vi "Main IU.vi"() -> ()   [LabVIEW 2018]
uses:
  <vilib>/Analysis/baseanly.llb/Mean (DBL).vi
  <vilib>/Utility/file.llb/Read Delimited Spreadsheet (DBL).vi
  <vilib>/Analysis/NI_AALBase.lvlib
panel:
  in  "Escriba el tiempo para ejecutar\ntrayectoria suave":dbl
  in  "Setpoint 2":dbl
  in  "Setpoint 1":dbl
  in  "Homing":bool
  out "EsfuerzoSat 2":dbl(graph)
  out "SetpointVsSalida 2":cluster{"Double":dbl, "Output":dbl}(graph)
  out "EsfuerzoSat":dbl(graph)
  out "SetpointVsSalida":cluster{"Double":dbl, "Output":dbl}(graph)
  out "Saving Data":bool
  in  "Record Button":bool
  in  "Filename":path=path "test.lvm"
  out "Motor1":waveform(dbl)[](graph)
  in  "Paro Emergencia:\nUI y RT":bool
  in  "Stop UI":bool
  # "s"
  # "Esta automáticamente se ejecutará"
  # "rad/s^2"
  # "rad/s^2"
  # "rad"
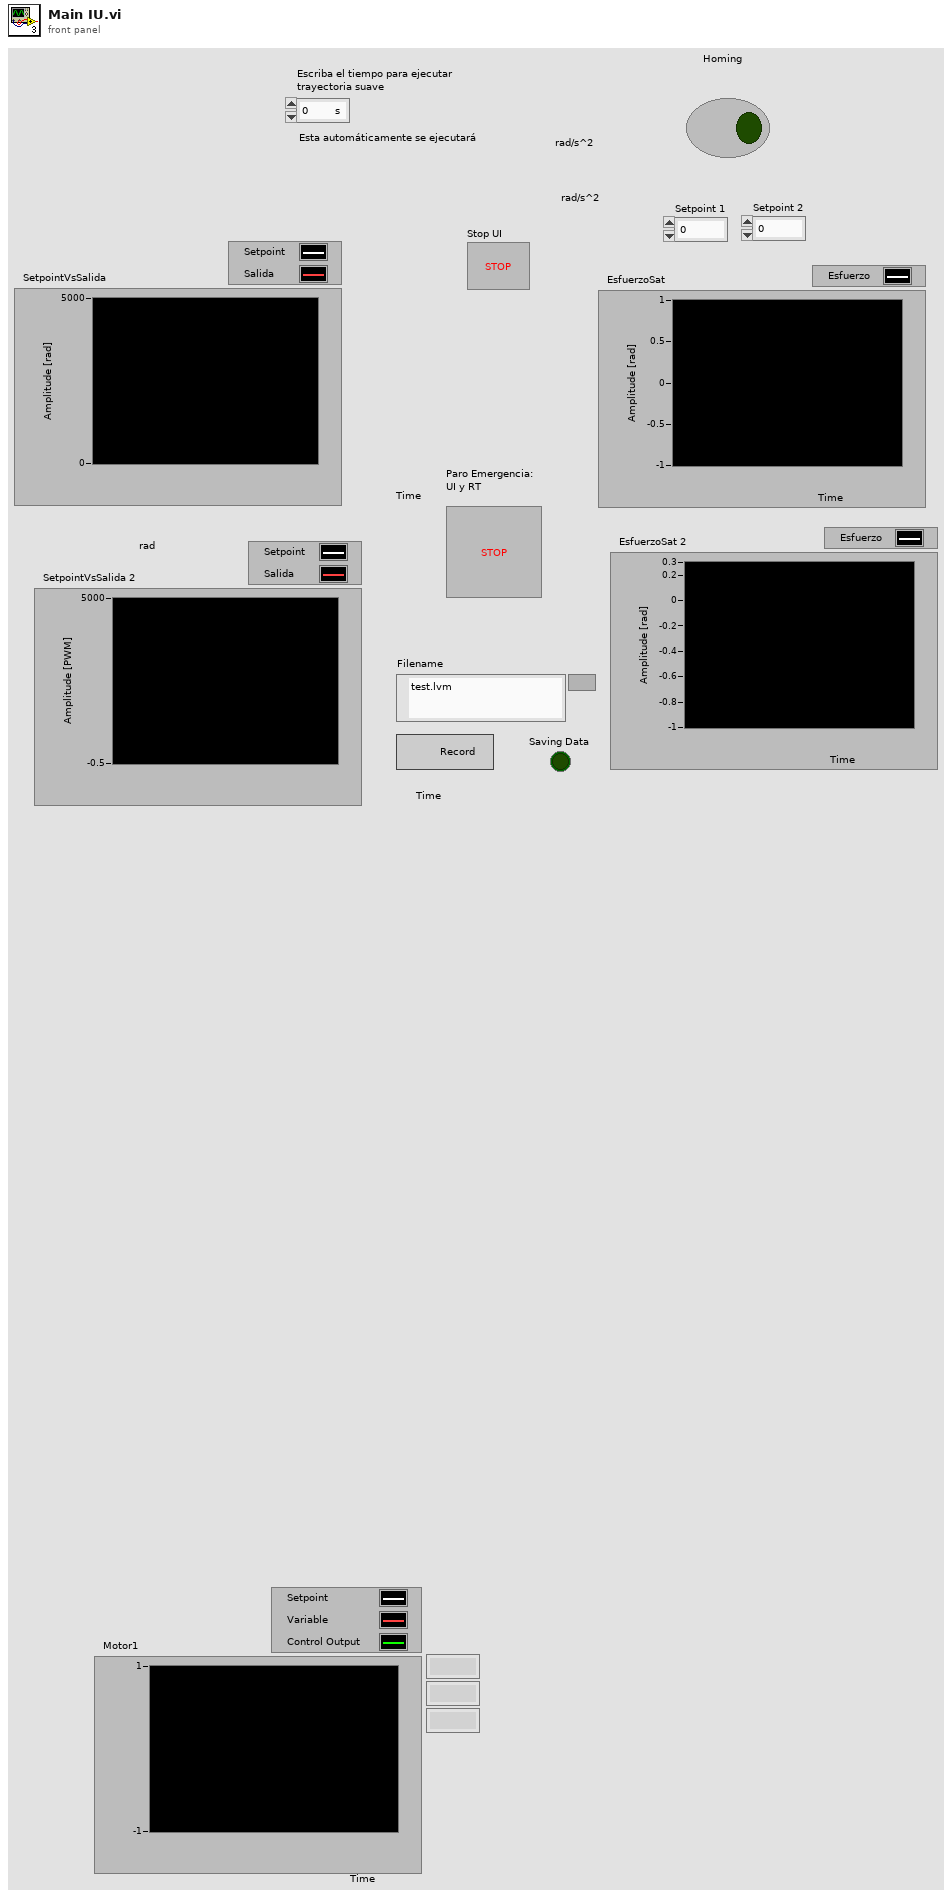
[diagram p1: front panel]
types:
  T1 = cluster{"Double":dbl, "dbl Scaled Value":dbl, "Output":dbl, "seconds since 1Jan1904":timestamp, dbl, dbl, dbl}
  T2 = cluster{"writer name":string, "Variant":variant, "Variant":variant}
  T3 = cluster{"Double":dbl, "dbl Scaled Value":dbl, "Output":dbl, "seconds since 1Jan1904":timestamp, dbl, dbl, dbl}[]
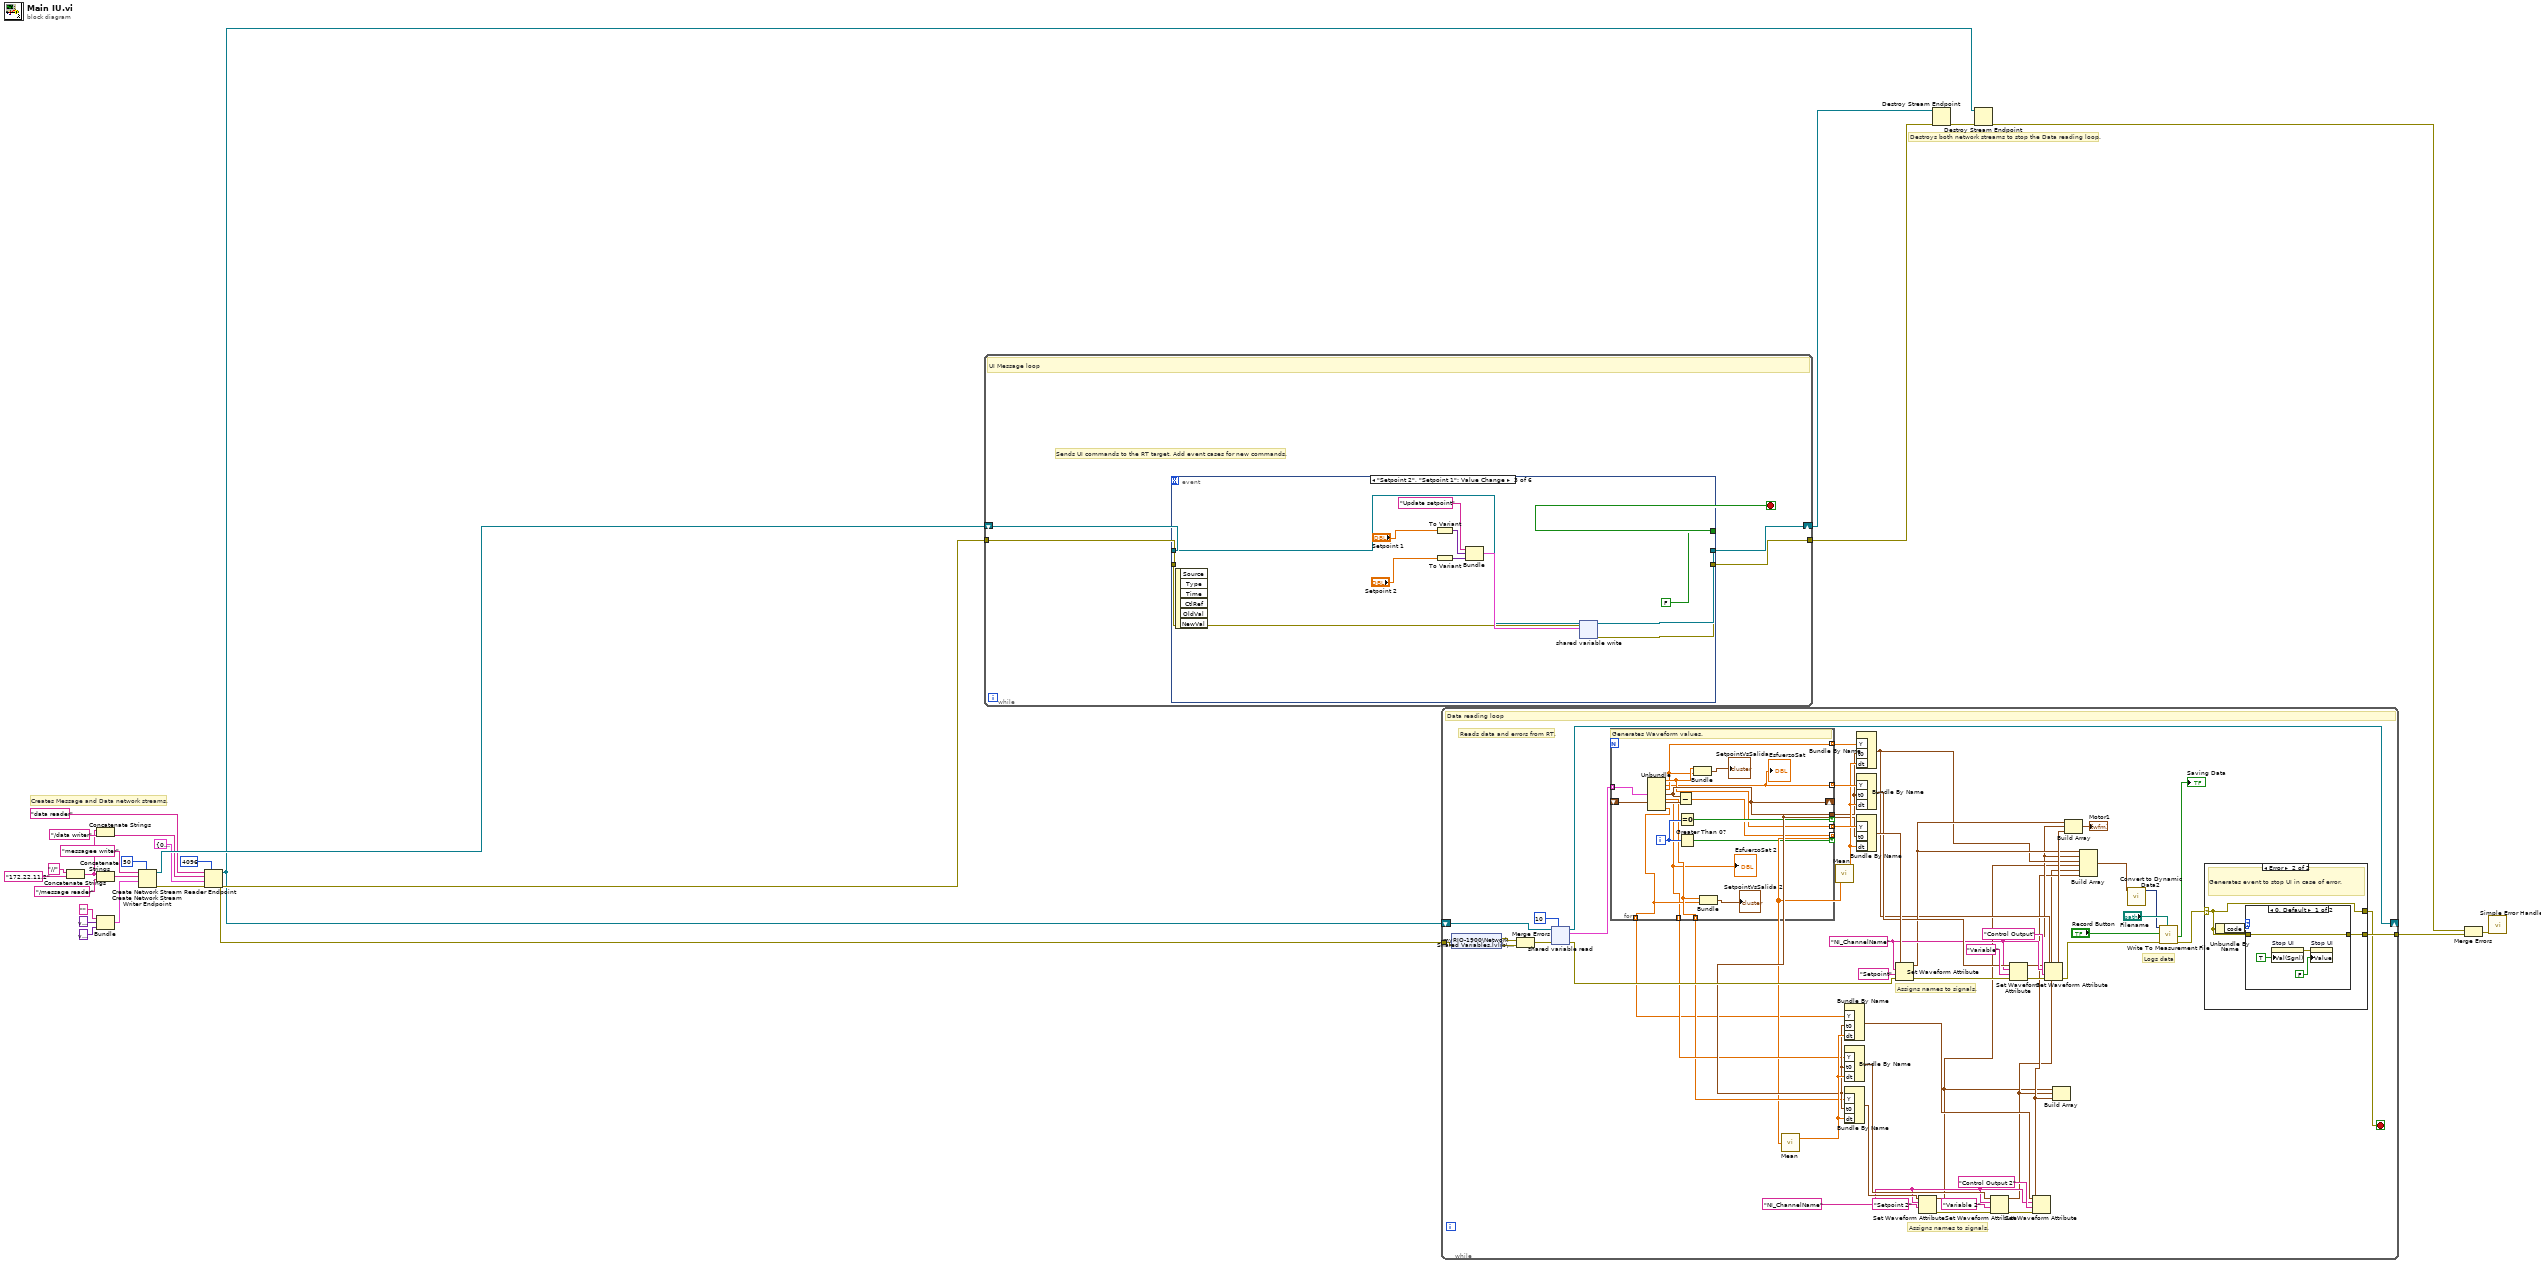
[diagram p0: block diagram]
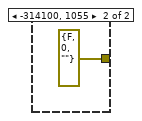
[diagram p3: hidden frame]
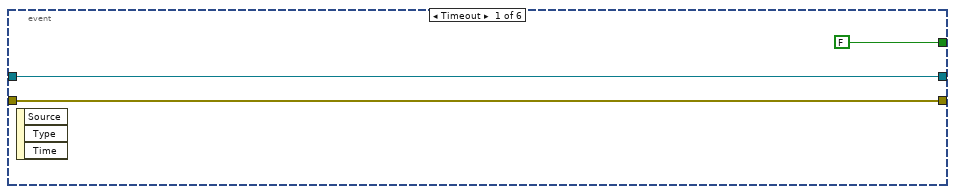
[diagram p4: hidden frame]
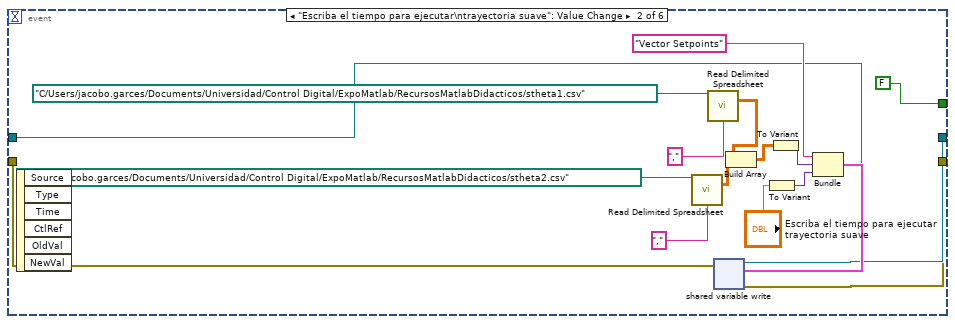
[diagram p5: hidden frame]
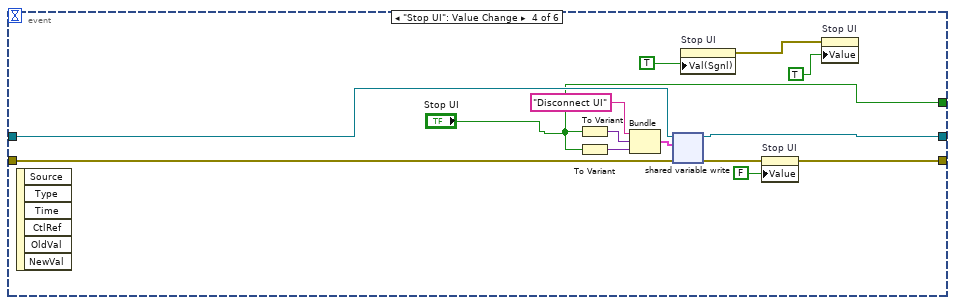
[diagram p6: hidden frame]
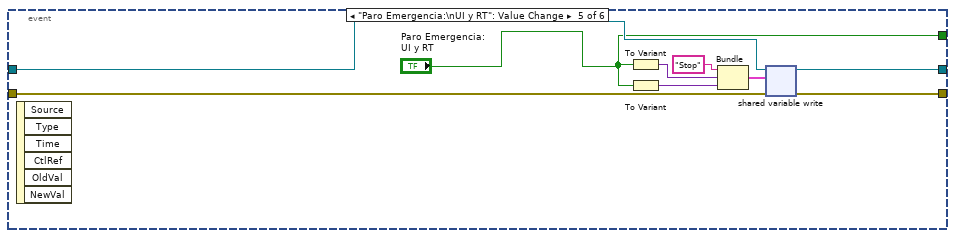
[diagram p7: hidden frame]
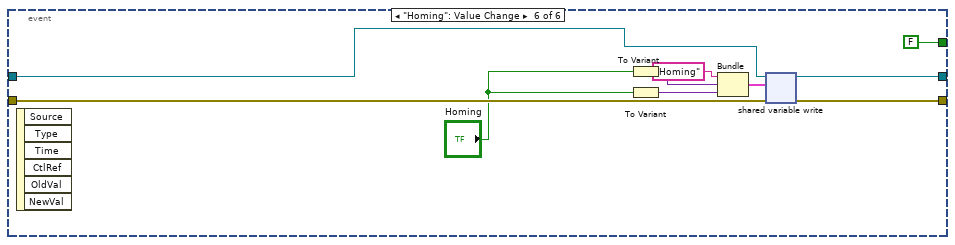
[diagram p8: hidden frame]
diagram:
  # "Destroys both network streams to stop the Data reading loop."
  # "Creates Message and Data network streams."
  n1 = Concatenate Strings("//", "172.22.11.2" ("myRIO IP")) -> (w2:string)
  n2 = Bundle("", variant, variant) -> (w26:cluster{string, variant, variant})  [unwired: 1 in]
  n3 = Concatenate Strings(w2, "/data writer") -> (w17:string)
  n4 = Concatenate Strings(w2, "/message reader") -> (w3:string)
  n5 = Create Network Stream Writer Endpoint(7:50 ("writer buffer size"), 9:w26, 10:w3, 11:"messagee writer" ("writer name")) -> (0:w14:errorcluster, 3:w20:refnum<k21>)  [unwired: 3 in]
  n6 = Create Network Stream Reader Endpoint(7:4096 ("reader buffer size"), 8:w14, 9:T1 {"Double"=0.0, "dbl Scaled Value"=0.0, "Output"=0.0, "seconds since 1Jan1904"=timestamp(0 s since 1904-01-01), 0.0, 0.0, 0.0} ("Data"), 10:w17, 11:"data reader" ("reader name")) -> (0:w13:errorcluster, 3:w6:refnum<k21>)  [unwired: 2 in]
  n7 = while {
    tunnel: w13 -> [w27]
    shift-right: [w31] -> w8
    shift-left: w20 -> [w28]
    tunnel: [w30] -> w9
    stop <- w29 stop-if-true
    # "Sends UI commands to the RT target. Add event cases for new commands."
    # "UI Message loop"
    n8 = event shown="[2] \"Setpoint 2\", \"Setpoint 1\": Value Change" {
      selector: _ -> [_ _ _ _ _ _]
      dyn-events: _ -> [_ _ _ _ _ _]
      timeout: _ -> [_ _ _ _ _ _]
      tunnel: [w33 w46 w57 w73 w81 w91] -> w31
      tunnel: [w32 w45 w56 w70 w82 w92] -> w30
      tunnel: [FALSE ("Stop UI and RT") FALSE ("Stop UI and RT") FALSE ("Stop UI and RT") "Stop UI" "Paro Emergencia:\nUI y RT" FALSE] -> w29
      tunnel: w28 -> [w33 w44 w55 w67 w79 w89]
      tunnel: w27 -> [w32 w43 w54 w68 w78 w88]
      event Timeout {
        n9 = event-data() -> ()  [unwired: 1 in, 3 out]
      }
      event "Escriba el tiempo para ejecutar\ntrayectoria suave": Value Change {
        n10 = event-data() -> ()  [unwired: 1 in, 6 out]
        n11 = call-poly <vilib>:"Read Delimited Spreadsheet.vi"("file path (dialog if empty)"=path "C:/Users/jacobo.garces/Documents/Universidad/Control Digital/ExpoMatlab/RecursosMatlabDidacticos/stheta2.csv", "delimiter (\\t)"="," ("delimiter (\\t)")) -> ("all rows"=w38:dbl[][])  [unwired: 8 in, 5 out]
        n12 = call-poly <vilib>:"Read Delimited Spreadsheet.vi"("file path (dialog if empty)"=path "C:/Users/jacobo.garces/Documents/Universidad/Control Digital/ExpoMatlab/RecursosMatlabDidacticos/stheta1.csv", "delimiter (\\t)"="," ("delimiter (\\t)")) -> ("all rows"=w37:dbl[][])  [unwired: 8 in, 5 out]
        n13 = Build Array(w37, w38) -> (w36:dbl[][][])
        n14 = To Variant(anything="Escriba el tiempo para ejecutar\ntrayectoria suave") -> (Variant=w49:variant)
        n15 = To Variant(anything=w36) -> (Variant=w47:variant)
        n16 = Bundle("writer name"="Vector Setpoints", "Variant"=w47, "Variant"=w49) -> (w48:T2)  [unwired: 1 in]
        n17 = shared-variable-write(w44, w43, w48) -> (w46:refnum<k21>, w45:errorcluster)  [unwired: 1 in, 1 out]
      }
      event "Setpoint 2", "Setpoint 1": Value Change {
        n18 = event-data() -> ()  [unwired: 1 in, 6 out]
        n19 = To Variant(anything="Setpoint 1") -> (Variant=w58:variant)
        n20 = To Variant(anything="Setpoint 2") -> (Variant=w60:variant)
        n21 = Bundle("writer name"="Update setpoint", "Variant"=w58, "Variant"=w60) -> (w59:T2)  [unwired: 1 in]
        n22 = shared-variable-write(w55, w54, w59) -> (w57:refnum<k21>, w56:errorcluster)  [unwired: 1 in, 1 out]
      }
      event "Stop UI": Value Change {
        n23 = event-data() -> ()  [unwired: 1 in, 6 out]
        n24 = To Variant(anything="Stop UI") -> (Variant=w76:variant)
        n25 = To Variant(anything="Stop UI") -> (Variant=w69:variant)
        n26 = Bundle("writer name"="Disconnect UI", "Variant"=w76, "Variant"=w69) -> (w75:T2)  [unwired: 1 in]
        n27 = shared-variable-write(w67, w68, w75) -> (w73:refnum<k21>, w71:errorcluster)  [unwired: 1 in, 1 out]
        n28 = property on="Stop UI" class="Bool (strict)"("Val(Sgnl)"=TRUE ("Stop UI and RT")) -> (error out=w66:errorcluster)  [unwired: 2 in, 1 out]
        n29 = property on="Stop UI" class="Bool (strict)"(error in=w71, "Value"=FALSE ("Stop UI and RT")) -> (error out=w70:errorcluster)  [unwired: 1 in, 1 out]
        n30 = property on="Stop UI" class="Bool (strict)"(error in=w66, "Value"=TRUE ("Stop UI")) -> ()  [unwired: 1 in, 2 out]
      }
      event "Paro Emergencia:\nUI y RT": Value Change {
        n31 = event-data() -> ()  [unwired: 1 in, 6 out]
        n32 = To Variant(anything="Paro Emergencia:\nUI y RT") -> (Variant=w85:variant)
        n33 = To Variant(anything="Paro Emergencia:\nUI y RT") -> (Variant=w80:variant)
        n34 = Bundle("writer name"="Stop", "Variant"=w85, "Variant"=w80) -> (w84:T2)  [unwired: 1 in]
        n35 = shared-variable-write(w79, w78, w84) -> (w81:refnum<k21>, w82:errorcluster)  [unwired: 1 in, 1 out]
      }
      event "Homing": Value Change {
        n36 = event-data() -> ()  [unwired: 1 in, 6 out]
        n37 = To Variant(anything="Homing") -> (Variant=w95:variant)
        n38 = To Variant(anything="Homing") -> (Variant=w90:variant)
        n39 = Bundle("writer name"="Homing", "Variant"=w95, "Variant"=w90) -> (w94:T2)  [unwired: 1 in]
        n40 = shared-variable-write(w89, w88, w94) -> (w91:refnum<k21>, w92:errorcluster)  [unwired: 1 in, 1 out]
      }
    }
  }
  n41 = while {
    tunnel: w13 -> [w123]
    shift-right: [w133] -> _
    shift-left: w6 -> [w148]
    tunnel: [w122] -> w10
    stop <- w121 stop-if-true
    w110 = "NI_ChannelName" ("name")
    w127 = "NI_ChannelName" ("name")
    # "Assigns names to signals."
    # "Logs data"
    # "Assigns names to signals."
    # "Reads data and errors from RT."
    # "Data reading loop"
    n42 = shared-variable "myRIO-1900\\Network Shared Variables.lvlib\\error IO"(error in=w123) -> (w126:errorcluster, error out=w125:errorcluster)
    n43 = Merge Errors(w126, w125) -> (w124:errorcluster)
    n44 = shared-variable-read(w148, w124, 10 ("# elements")) -> (w133:refnum<k21>, w138:errorcluster, w146:T3)  [unwired: 1 in, 1 out]
    n45 = for {
      tunnel: w146 -> [w172] mode=indexing
      tunnel: [w165] -> w145 mode=indexing
      tunnel: [w162] -> w144 mode=indexing
      tunnel: [w164] -> w120 mode=indexing
      tunnel: [w170] -> w109 if=w171
      shift-right: [w170] -> _
      shift-left: _ -> [w169]
      tunnel: [w168] -> w106 mode=indexing if=w166
      tunnel: [w159] -> w105 mode=indexing
      tunnel: [w158] -> w108 mode=indexing
      tunnel: [w160] -> w107 mode=indexing
      i -> [w167]
      # "Generates Waveform values."
      n46 = Unbundle(w172) -> ("Double"=w165:dbl, "dbl Scaled Value"=w162:dbl, "Output"=w164:dbl, "seconds since 1Jan1904"=w170:timestamp, w160:dbl, w158:dbl, w159:dbl)
      "EsfuerzoSat" <- w162
      "EsfuerzoSat 2" <- w158
      n47 = Subtract(x=w170, y=w169) -> (x-y=w168:dbl)
      n48 = Equal To 0?(x=w167) -> (x = 0?=w171:bool)
      n49 = Greater Than 0?(x=w167) -> (x > 0?=w166:bool)
      n50 = Bundle("Double"=w165, "Output"=w164) -> (→"SetpointVsSalida":cluster{"Double":dbl, "Output":dbl})  [unwired: 1 in]
      n51 = Bundle(w160, w159) -> (→"SetpointVsSalida 2":cluster{dbl, dbl})  [unwired: 1 in]
    }
    n52 = call-poly <vilib>:"Mean.vi"("X"=w106) -> ("mean"=w119:dbl)  [unwired: 1 out]
    n53 = call-poly <vilib>:"Mean.vi"("X"=w106) -> ("mean"=w143:dbl)  [unwired: 1 out]
    n54 = Bundle By Name("Y"=w105, "t0"=w109, "dt"=w119) -> (w111:waveform(dbl))  [unwired: 1 in]
    n55 = Bundle By Name("Y"=w108, "t0"=w109, "dt"=w119) -> (w112:waveform(dbl))  [unwired: 1 in]
    n56 = Bundle By Name("Y"=w107, "t0"=w109, "dt"=w119) -> (w118:waveform(dbl))  [unwired: 1 in]
    n57 = Bundle By Name("Y"=w120, "t0"=w109, "dt"=w143) -> (w101:waveform(dbl))  [unwired: 1 in]
    n58 = Bundle By Name("Y"=w144, "t0"=w109, "dt"=w143) -> (w135:waveform(dbl))  [unwired: 1 in]
    n59 = Bundle By Name("Y"=w145, "t0"=w109, "dt"=w143) -> (w142:waveform(dbl))  [unwired: 1 in]
    n60 = Set Waveform Attribute(4:w138, 5:"Setpoint" ("name"), 6:w127, 7:w142) -> (0:w137:errorcluster, 3:w102:waveform(dbl))  [unwired: 1 out]
    n61 = Set Waveform Attribute(5:"Setpoint 2" ("name"), 6:w110, 7:w118) -> (0:w114:errorcluster, 3:w97:waveform(dbl))  [unwired: 1 in, 1 out]
    n62 = Set Waveform Attribute(4:w114, 5:"Variable 2" ("name"), 6:w110, 7:w112) -> (0:w113:errorcluster, 3:w98:waveform(dbl))  [unwired: 1 out]
    n63 = Set Waveform Attribute(4:w137, 5:"Variable" ("name"), 6:w127, 7:w135) -> (0:w136:errorcluster, 3:w100:waveform(dbl))  [unwired: 1 out]
    n64 = Set Waveform Attribute(4:w113, 5:"Control Output 2" ("name"), 6:w110, 7:w111) -> (3:w99:waveform(dbl))  [unwired: 2 out]
    n65 = Set Waveform Attribute(4:w136, 5:"Control Output" ("name"), 6:w127, 7:w101) -> (0:w132:errorcluster, 3:w134:waveform(dbl))  [unwired: 1 out]
    n66 = Build Array(w97, w98, w99) -> ()  [unwired: 1 out]
    n67 = Build Array(w102, w100, w134) -> (→"Motor1":waveform(dbl)[])
    n68 = Build Array(w102, w100, w101, w97, w98, w99) -> (w96:waveform(dbl)[])
    n69 = call "Convert to Dynamic Data2"("Array of Waveforms"=w96) -> ("Dynamic Data Type"=w103:dynamicdata)  [unwired: 3 in]
    n70 = call "Write To Measurement File"("Signals"=w103, "Enable"="Record Button", "error in (no error)"=w132, "Filename"="Filename") -> ("Saving Data"=→"Saving Data":bool, "error out"=w128:errorcluster)  [unwired: 13 in, 1 out]
    n71 = case shown="Error" w128 {
      selector: w128 -> [w149 w150]
      tunnel: [w149 w151] -> w122
      tunnel: [w149 w150] -> w121
      frame No Error {
        # "No action required."
      }
      frame Error {
        # "Generates event to stop UI in case of error."
        n72 = Unbundle By Name(w150) -> ("code"=w152:i32)
        n73 = case shown="0, Default" w152 {
          tunnel: [w155 errorcluster {"status"=FALSE, "code"=0, "source"=""} ("error IO")] -> w151
          tunnel: w150 -> [w155 _]
          frame 0, Default {
            n74 = property on="Stop UI" class="Bool (strict)"("Val(Sgnl)"=TRUE ("Stop UI and RT")) -> (error out=w154:errorcluster)  [unwired: 2 in, 1 out]
            n75 = property on="Stop UI" class="Bool (strict)"(error in=w154, "Value"=FALSE ("Stop UI")) -> ()  [unwired: 1 in, 2 out]
          }
          frame -314100, 1055 {
          }
        }
      }
    }
  }
  n76 = Destroy Stream Endpoint(8:w9, 11:w8) -> (0:w7:errorcluster)
  n77 = Destroy Stream Endpoint(8:w7, 11:w6) -> (0:w5:errorcluster)
  n78 = Merge Errors(w5, w10) -> (w11:errorcluster)
  n79 = call <vilib>:"Simple Error Handler.vi"("error in (no error)"=w11) -> ()  [unwired: 4 in, 5 out]
